vi "ni579x Wait for Initialization.vi"(0 "Register Bus":T1, 9 "timeout [s]":dbl=15.0, 11 "Error In":errorcluster) -> (4 "Register Bus (out)":T1, 15 "Error Out":errorcluster)   [LabVIEW 2015, in "ni579x Config v2 Host.lvlib"]
uses:
  <instrlib>/ni579x/Config/v2/Host/ni579x Config v2 Host.lvlib
  <instrlib>/_niInstr/Register Bus/v0/Host/Public/Register Bus Session.ctl
  <instrlib>/_niInstr/Register Bus/v0/Host/Private/Session Data.ctl
  <instrlib>/ni579x/Config/v2/Shared/Types/ni579x Required FPGA Interface Reference.ctl
  <vilib>/Utility/error.llb/Error Cluster From Error Code.vi
  <vilib>/rvi/errors/niLvFpgaAdjustHostInterfaceError.vi
  <vilib>/rvi/interface/nirviReadWriteControl/nirviReadWriteControl.xnode
  <instrlib>/ni579x/Config/v2/Shared/ni579x Config v2 Shared.lvlib
  NiFpgaLv.dll
  <vilib>/rvi/interface/Simulation/niFpgaSimulationCallBeginRW.vi
  <instrlib>/_niInstr/Register Bus/v0/Host/niInstr Register Bus v0 Host.lvlib
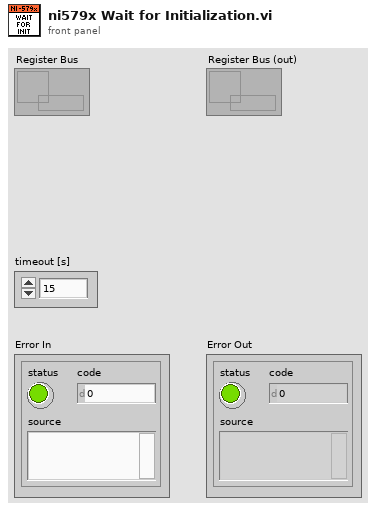
[diagram p1: front panel]
types:
  T1 = typedef "niInstr Register Bus v0 Host.lvlib/Register Bus Session.ctl" = refnum<queue>
  T2 = typedef "ni579x Config v2 Shared.lvlib/ni579x Required FPGA Interface Reference.ctl" = refnum<k20>
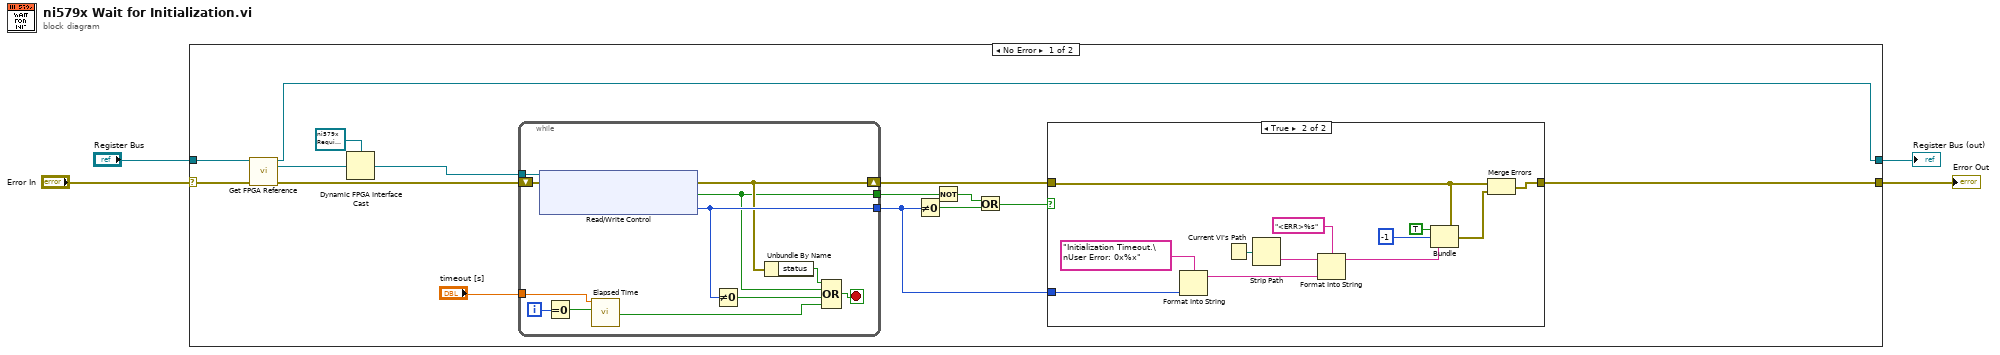
[diagram p0: block diagram]
diagram:
  n1 = case shown="No Error" "Error In" {
    selector: "Error In" -> [w18 w46]
    tunnel: [w7 w46] -> w3
    tunnel: "Register Bus" -> [w19 w45]
    tunnel: [w6 w45] -> w1
    frame No Error {
      n2 = call <instrlib>:"Get FPGA Reference.vi"("session in"=w19, "error in"=w18) -> ("session out"=w6:T1, "fpga ref"=w17:refnum<k20>, "error out"=w9:errorcluster)  [unwired: 11 in]
      n3 = Dynamic FPGA Interface Cast(Session In=T2 refnum ("Type"), Type=w17) -> (Session Out=w8:T2)
      n4 = while {
        tunnel: w8 -> [w37]
        tunnel: [w33] -> w16
        shift-right: [w34] -> w12
        shift-left: w9 -> [w35]
        tunnel: [w36] -> w11
        tunnel: "timeout [s]" -> [w38]
        i -> [w43]
        stop <- w41 stop-if-true
        n5 = xnode "Read/Write Control"("FPGA VI Reference In"=w37, "error in"=w35) -> ("error out"=w34:errorcluster, "IO Module\\Initialization Done"=w33:bool, "IO Module\\User Error"=w36:u8)  [unwired: 1 out]
        n6 = Equal To 0?(x=w43) -> (x = 0?=w44:bool)
        n7 = call "Elapsed Time"("Time Target (s)"=w38, "Reset"=w44) -> ("Time has Elapsed"=w42:bool)  [unwired: 10 in, 7 out]
        n8 = Not Equal To 0?(x=w36) -> (x != 0?=w39:bool)
        n9 = Unbundle By Name(w34) -> ("status"=w40:bool)
        n10 = Compound Arithmetic op=OR(w40, w33, w39, w42) -> (w41:bool)
      }
      n11 = Not Equal To 0?(x=w11) -> (x != 0?=w14:bool)
      n12 = Not(x=w16) -> (.not. x?=w15:bool)
      n13 = Or(x=w15, y=w14) -> (x .or. y?=w13:bool)
      n14 = case shown="True" w13 {
        tunnel: w12 -> [w20 w24]
        tunnel: [w20 w21] -> w7
        tunnel: w11 -> [_ w22]
        frame False {
        }
        frame True {
          n15 = Format Into String(format string="Initialization Timeout.\nUser Error: 0x%x" ("error message (\"\")"), w22) -> (resulting string=w23:string)  [unwired: 2 in, 1 out]
          n16 = Current VI's Path() -> (path=w30:path)
          n17 = Strip Path(path=w30) -> (name=w29:string)  [unwired: 1 out]
          n18 = Format Into String(format string="<ERR>%s", initial string=w29, w23) -> (resulting string=w28:string)  [unwired: 1 in, 1 out]
          n19 = Bundle(cluster=w24, "status"=TRUE, "code"=-1, "source"=w28) -> (w27:errorcluster)
          n20 = Merge Errors(w24, w27) -> (w21:errorcluster)
        }
      }
    }
    frame Error {
    }
  }
  "Register Bus (out)" <- w1
  "Error Out" <- w3
